vi "findNewLocationV2.vi"(8 "error in (no error)":errorcluster, 9 "possible \nlocations":dbl[](array[numeric]), 11 "goal location":dbl) -> (0 "error out":errorcluster, 3 "new\nplatform":i32)   [LabVIEW 2017]
panel:
  out "DAQmx Channel":string
  # "V2 determines when animal reaches the goal location\n\nV1 determines when animal no longer at start location"
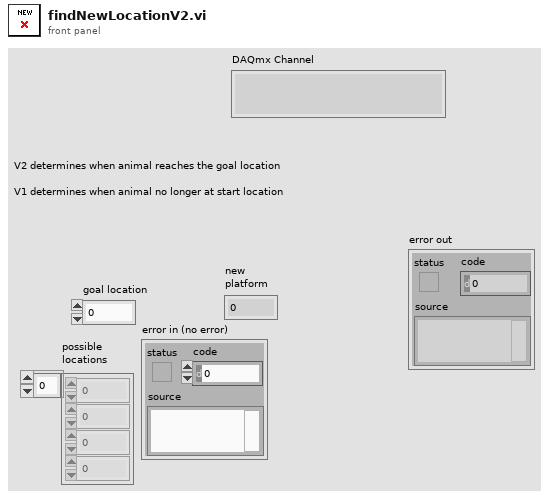
[diagram p1: front panel]
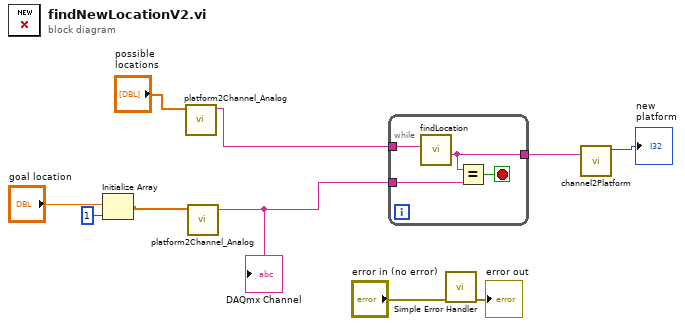
[diagram p0: block diagram]
diagram:
  n1 = Initialize Array("goal location", 1 ("dimension size")) -> (w1:dbl[])
  n2 = call "platform2Channel_Analog.vi"("platforms"="possible \nlocations") -> ("DAQmx Channel"=w10:string)  [unwired: 10 in]
  n3 = call "platform2Channel_Analog.vi"("platforms"=w1) -> ("DAQmx Channel"=w8:string)  [unwired: 10 in]
  "DAQmx Channel" <- w8
  n4 = while {
    tunnel: w8 -> [w13]
    tunnel: [w12] -> w7
    tunnel: w10 -> [w11]
    stop <- w14 stop-if-true
    n5 = call "findLocation.vi"("DAQmx \nPhysical Channel"=w11) -> ("Animals location"=w12:string)  [unwired: 10 in]
    n6 = Equal?(x=w12, y=w13) -> (x = y?=w14:bool)
  }
  n7 = call <vilib>:"Simple Error Handler.vi"("error in (no error)"="error in (no error)") -> ("error out"=→"error out":errorcluster)  [unwired: 4 in, 4 out]
  n8 = call "channel2Platform.vi"("DAQmx \nPhysical Channel"=w7) -> ("Platform number"=→"new\nplatform":i32)  [unwired: 10 in]
